vi "Initiate from Array.vi"(8 "error in (no error)":errorcluster, 10 "Prefix Array":string[](array[string]), 11 "Array":variant[](array[variant])) -> (0 "error out":errorcluster, 3 "ClusterTree out":refnum<class "TreeLUT.lvclass">)   [LabVIEW 2017, in "TreeLUT.lvclass"]
uses:
  TreeLUT.lvclass
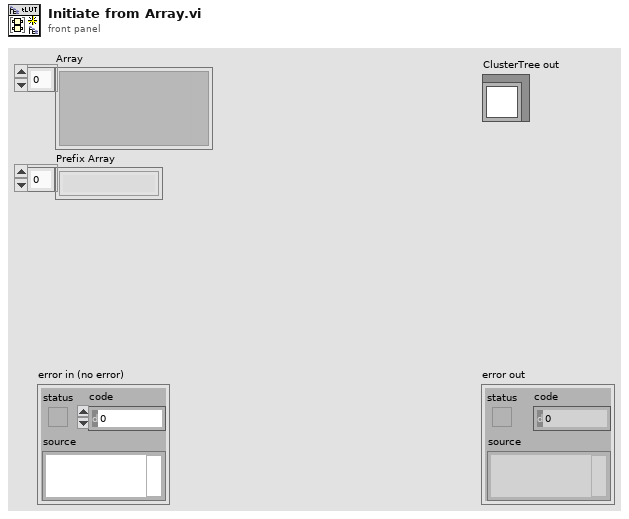
[diagram p1: front panel]
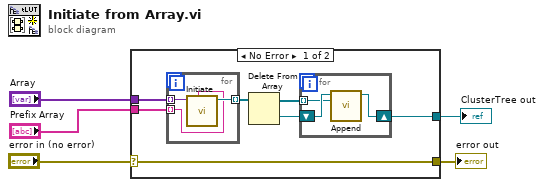
[diagram p0: block diagram]
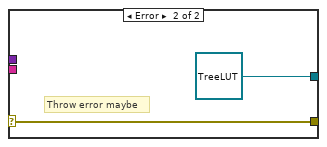
[diagram p2: hidden frame]
diagram:
  n1 = case shown="No Error" "error in (no error)" {
    selector: "error in (no error)" -> [w12 w20]
    tunnel: [w12 w20] -> w4
    tunnel: "Array" -> [w11 _]
    tunnel: [w7 refnum<class "TreeLUT.lvclass"> refnum ("ClusterTree out")] -> w2
    tunnel: "Prefix Array" -> [w6 _]
    frame No Error {
      n2 = for {
        tunnel: w11 -> [w18] mode=indexing
        tunnel: [w17] -> w10 mode=indexing
        tunnel: w6 -> [w16] mode=indexing
        n3 = call "Initiate.vi"("If Empty"=w16, "Raw Variant"=w18) -> ("ClusterTree out"=w17:refnum<class "TreeLUT.lvclass">)  [unwired: 8 in, 1 out]
      }
      n4 = Delete From Array(array=w10) -> (deleted portion=w8:refnum<class "TreeLUT.lvclass">, array with subset deleted=w9:refnum<class "TreeLUT.lvclass">[])  [unwired: 2 in]
      n5 = for {
        tunnel: w9 -> [w14] mode=indexing
        shift-right: [w13] -> w7
        shift-left: w8 -> [w15]
        n6 = call "Append.vi"("ClusterTree to Append"=w14, "ClusterTree In"=w15) -> ("ClusterTree out"=w13:refnum<class "TreeLUT.lvclass">)  [unwired: 8 in, 1 out]
      }
    }
    frame Error {
      # "Throw error maybe"
    }
  }
  "error out" <- w4
  "ClusterTree out" <- w2
